vi "Init Actor Layer.vi"() -> (5 "Actor Layer":refnum<class "Actor Layer.lvclass">)   [LabVIEW 2020, in "_Template.lvlib" / "{{Actor}}.lvlib"]
uses:
  {{Actor}}.lvlib
  jettl/jettl/Actor Layer/Actor Layer.lvclass
  Actor Layer/Actor Layer.lvclass
  C:/Users/nathan.davis/Desktop/personal/jettl-harness/repos/jettl/src/jettl/jettl/Actor Layer/Actor Layer.lvclass
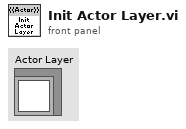
[diagram p1: front panel]
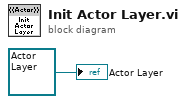
[diagram p0: block diagram]
diagram:
  "Actor Layer" <- refnum<class "Actor Layer.lvclass"> refnum ("_Template.lvlib:{{Actor}}.lvlib:Actor.lvclass")
